vi "Define_Matrices.vi"() -> ()   [LabVIEW 2020]
uses:
  <vilib>/Analysis/Matrix/Datatypes/RealMatrix.ctl
  <vilib>/Analysis/Matrix/NI_Matrix.lvlib
panel:
  out "G Matrix":T1
  out "Q = GQG'":T1
  out "R Matrix":T1=[[1e-10, 0.0], [0.0, 1e-11]]
  in  "Sampling Freqauency (Hz)":dbl=10000.0
  out "F  Matrix":T1=[[1.0, 0.0001], [0.0, 1.0]]
  out "H Matrix":T1=[[0.0, 1.0], [9.81, 0.0]]
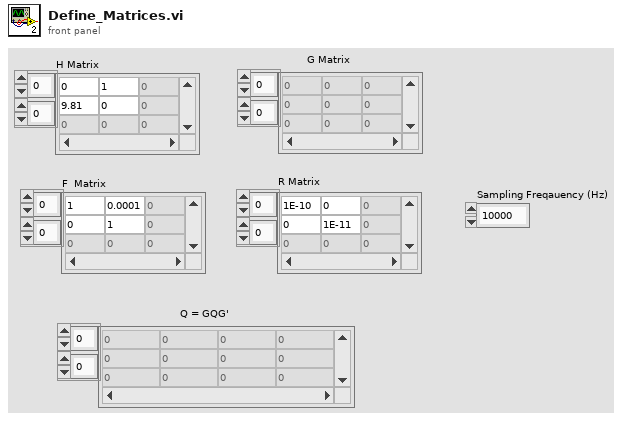
[diagram p1: front panel]
types:
  T1 = typedef "NI_Matrix.lvlib/RealMatrix.ctl" = dbl[][]
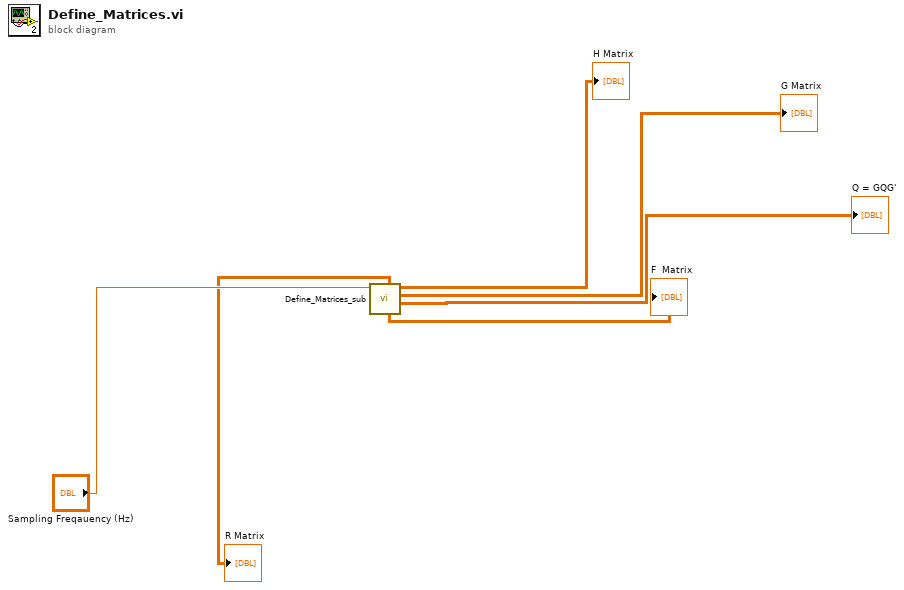
[diagram p0: block diagram]
diagram:
  n1 = call "Define_Matrices_sub.vi"("Sampling Freqauency (Hz)"="Sampling Freqauency (Hz)") -> ("Q = GQG'"=→"Q = GQG'":T1, "G Matrix"=→"G Matrix":T1, "H Matrix"=→"H Matrix":T1, "F  Matrix"=→"F  Matrix":T1, "R Matrix"=→"R Matrix":T1)  [unwired: 6 in]
